vi "Create Channel Configuration.vi"(4 "non-random type (DBL)":T1=enum."DBL", 6 "random types? (F)":bool, 7 "base channel name (channel)":string="channel", 11 "channel count":i32) -> (2 "buffer size":u64, 3 "channel configurations":T2[](array[typedef]))   [LabVIEW 2017]
uses:
  Source/Shared/Typedefs/DSF.Shared.Refactor.Typedefs.Channel Array Configuration.ctl
  Source/Shared/Typedefs/DSF.Shared.Typedefs.Data Type.ctl
  Source/Shared/VIs/DSF.Shared.Data Type.Sizeof.vi
  Source/DSF.Shared.lvlib
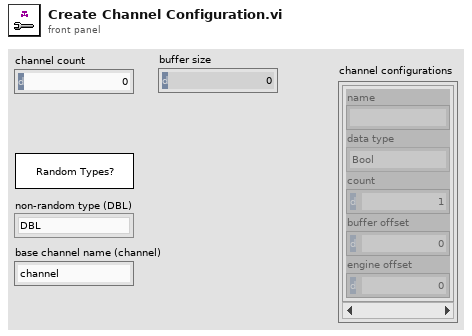
[diagram p1: front panel]
types:
  T1 = typedef "DSF.Shared.lvlib/DSF.Shared.Typedefs.Data Type.ctl" = enum8{"Bool", "SGL", "DBL", "I8", "I16", "I32", "I64", "U8", "U16", "U32", "U64"}
  T2 = typedef "DSF.Shared.lvlib/DSF.Shared.Refactor.Typedefs.Channel Array Configuration.ctl" = cluster{"name":string, "data type":T1, "count":u64, "buffer offset":u64, "engine offset":u64}
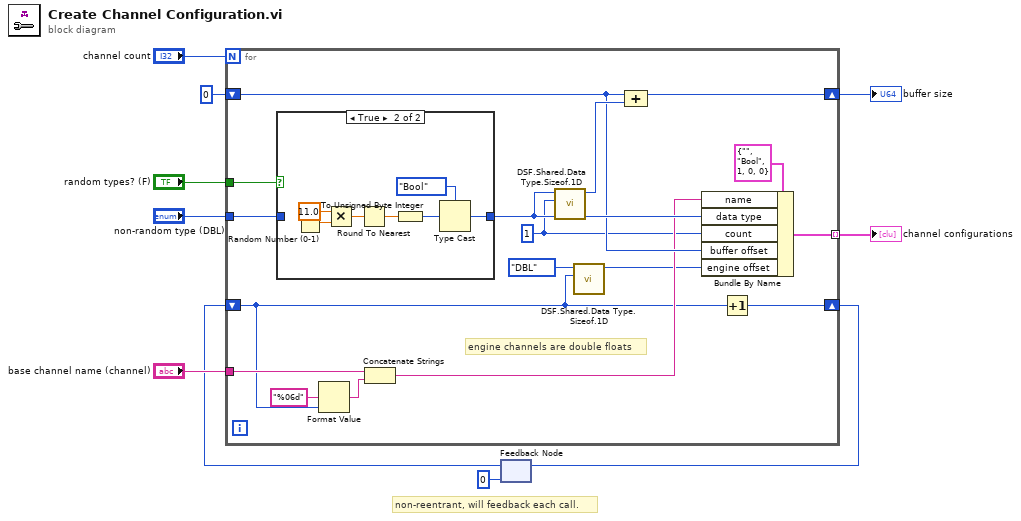
[diagram p0: block diagram]
diagram:
  # "non-reentrant, will feedback each call."
  n1 = feedback #1(u64 0) -> (w3:u64)
  n2 = for {
    N: "channel count" -> [_]
    tunnel: "non-random type (DBL)" -> [w25]
    tunnel: "random types? (F)" -> [w26]
    shift-right: [w23] -> w4
    shift-left: u64 0 ("buffer offset") -> [w21]
    tunnel: "base channel name (channel)" -> [w18]
    tunnel: [w16] -> w5 mode=indexing
    shift-right: [w14] -> w1
    shift-left: w3 -> [w12]
    w13 = u64 1 ("count")
    # "engine channels are double floats"
    n3 = case shown="True" w26 {
      tunnel: [w28 w29] -> w24
      tunnel: w25 -> [w28 _]
      frame False {
      }
      frame True {
        n4 = Random Number (0-1)() -> (number: 0 to 1=w34:dbl)
        n5 = Multiply(x=11.0, y=w34) -> (x*y=w30:dbl)
        n6 = Round To Nearest(number=w30) -> (nearest integer value=w35:dbl)
        n7 = To Unsigned Byte Integer(number=w35) -> (unsigned 8bit integer=w32:u8)
        n8 = Type Cast(type=DSF.Shared.Typedefs.Data_Type."Bool" ("data type"), x=w32) -> (*(type *) &x=w29:T1)
      }
    }
    n9 = Format Value(format string="%06d", value (0)=w12) -> (output string=w20:string)  [unwired: 1 in]
    n10 = Concatenate Strings(w18, w20) -> (w17:string)
    n11 = call "DSF.Shared.Data Type.Sizeof.1D.vi"("count"=w13, "data type"=w24) -> ("size in bytes"=w22:u64)  [unwired: 9 in]
    n12 = call "DSF.Shared.Data Type.Sizeof.1D.vi"("count"=w12, "data type"=DSF.Shared.Typedefs.Data_Type."DBL") -> ("size in bytes"=w11:u64)  [unwired: 9 in]
    n13 = Compound Arithmetic op=ADD(w21, w22) -> (w23:u64)
    n14 = Bundle By Name(cluster=T2 {"name"="", "data type"=enum."Bool", "count"=1, "buffer offset"=0, "engine offset"=0} ("Channel Configuration"), "name"=w17, "data type"=w24, "count"=w13, "buffer offset"=w21, "engine offset"=w11) -> (w16:T2)
    n15 = Increment(x=w12) -> (x+1=w14:u64)
  }
  "channel configurations" <- w5
  "buffer size" <- w4
  n16 = feedback-in #1(w1) -> ()
